vi "SQLite Add Cycle Test.vi"(7 "Test DB Set Up Command":string, 8 "Error In (no error)":errorcluster, 11 "SQLite DB Operator In":refnum<class "SQLite DB Operator.lvclass">) -> (0 "Error Out":errorcluster, 3 "SQLite DB OperatorOut":refnum<class "SQLite DB Operator.lvclass">)   [LabVIEW 2023]
uses:
  Clasess/SQLite DB Operator/SQLite DB Operator.lvclass
  Clasess/DB Records/Expenses Tracker Cycle/Public/Ctrls/Cycle.ctl
  Clasess/DB Records/Expenses Tracker Cycle/Expenses Tracker Cycle.lvclass
  H:/Desktop/LabVIEW/LabView Repo/Expenses-Tracker-DB-Operator/Interfaces/Expenses Tracker Record/Expenses Tracker Record.lvclass
  <vilib>/drjdpowell/SQLite Library/SQL Connection/Execute SQL (1D Cluster).vi
  <vilib>/addons/_JKI Toolkits/Caraya/classes/Test/Test.lvclass
  <vilib>/drjdpowell/SQLite Library/SQLite.lvlib
  H:/Desktop/LabVIEW/LabView Repo/Expenses-Tracker-DB-Operator/Clasess/DB Records/Expenses Tracker Cycle/Expenses Tracker Cycle.lvclass
  <vilib>/drjdpowell/SQLite Library/SQL Connection/Connection.lvclass
  Support/Adding/Add Record Assert Error.vi
  Support/Adding/Add Record Assert Not Error.vi
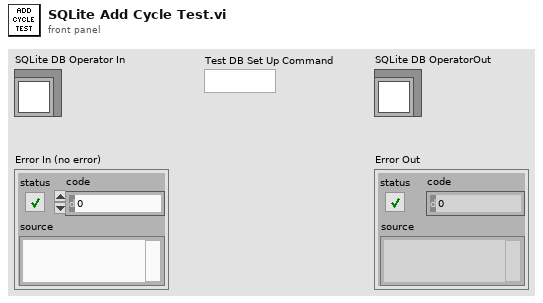
[diagram p1: front panel]
types:
  T1 = typedef "Expenses Tracker Cycle.lvclass/Cycle.ctl" = cluster{"ID":u32, "Name":string, "Day_of_occurence":u8, "Description":string}
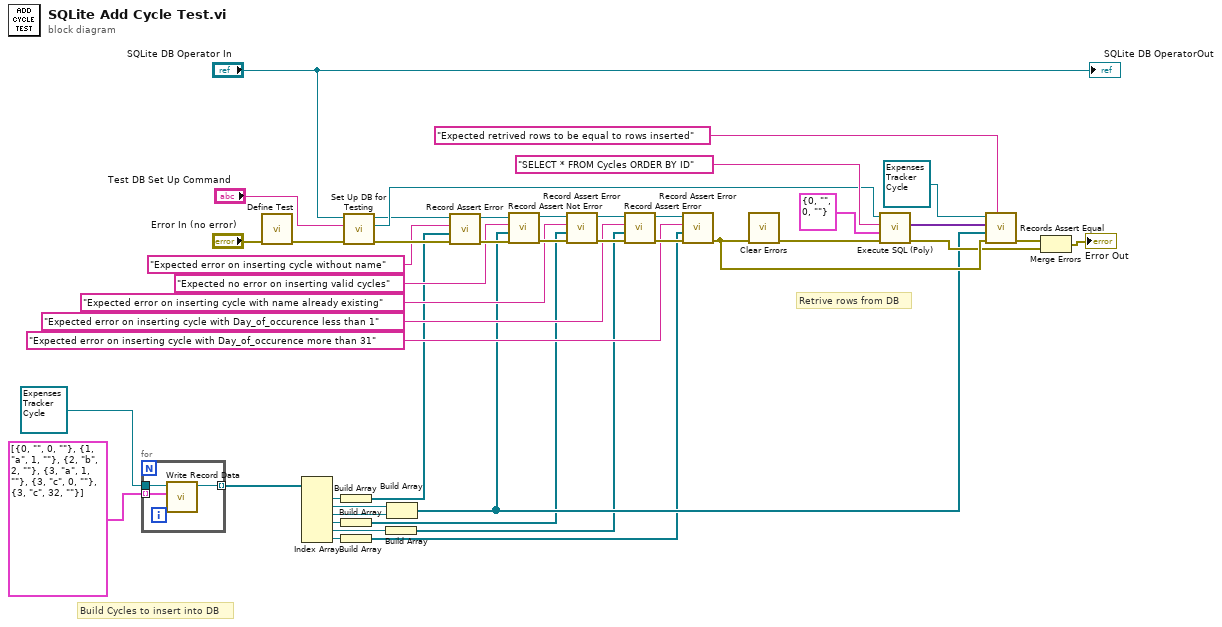
[diagram p0: block diagram]
diagram:
  # "Retrive rows from DB"
  # "Build Cycles to insert into DB"
  n1 = for {
    tunnel: T1[] [{"ID"=0, "Name"="", "Day_of_occurence"=0, "Description"=""}, {"ID"=1, "Name"="a", "Day_of_occurence"=1, "Description"=""}, {"ID"=2, "Name"="b", "Day_of_occurence"=2, "Description"=""}, {"ID"=3, "Name"="a", "Day_of_occurence"=1, "Description"=""}, {"ID"=3, "Name"="c", "Day_of_occurence"=0, "Description"=""}, {"ID"=3, "Name"="c", "Day_of_occurence"=32, "Description"=""}] ("Array") -> [w47] mode=indexing
    tunnel: refnum<class "Expenses Tracker Cycle.lvclass"> refnum ("Expenses Tracker Category") -> [w46]
    tunnel: [w45] -> w41 mode=indexing
    n2 = call-dynamic "Write Record Data.vi"("Record"=w47, "Expenses Tracker Cycle In"=w46) -> ("Expenses Tracker Cycle Out"=w45:refnum<class "Expenses Tracker Cycle.lvclass">)  [unwired: 8 in, 1 out]
  }
  n3 = call <vilib>:"Define Test.vi"("error in (no error)"="Error In (no error)") -> ("error out"=w32:errorcluster)  [unwired: 9 in, 1 out]
  n4 = Index Array(array=w41) -> (element #1=w40:refnum<class "Expenses Tracker Cycle.lvclass">, element #2=w39:refnum<class "Expenses Tracker Cycle.lvclass">, element #3=w38:refnum<class "Expenses Tracker Cycle.lvclass">, element #4=w6:refnum<class "Expenses Tracker Cycle.lvclass">, element #5=w4:refnum<class "Expenses Tracker Cycle.lvclass">, element #6=w35:refnum<class "Expenses Tracker Cycle.lvclass">)  [unwired: 6 in]
  n5 = Build Array(w40) -> (w8:refnum<class "Expenses Tracker Cycle.lvclass">[])
  n6 = Build Array(w6) -> (w5:refnum<class "Expenses Tracker Cycle.lvclass">[])
  n7 = Build Array(w35) -> (w1:refnum<class "Expenses Tracker Cycle.lvclass">[])
  n8 = call "Set Up DB for Testing.vi"("Error In (no error)"=w32, "Test DB Set Up Command"="Test DB Set Up Command", "SQLite DB Operator In"="SQLite DB Operator In") -> ("Error Out"=w31:errorcluster, "SQLite Connection"=w34:refnum<class "Connection.lvclass">, "SQLite DB Operator Out"=w30:refnum<class "SQLite DB Operator.lvclass">)  [unwired: 6 in]
  n9 = Build Array(w4) -> (w3:refnum<class "Expenses Tracker Cycle.lvclass">[])
  n10 = Build Array(w39, w38) -> (w7:refnum<class "Expenses Tracker Cycle.lvclass">[])
  n11 = call-poly "Record Assert Error.vi"("Error In"=w31, "Records"=w8, "Assertion Label"="Expected error on inserting cycle without name" ("Label (VI Title)"), "SQLite DB Operator In"=w30) -> ("Error Out"=w22:errorcluster, "SQLite DB Operator Out"=w21:refnum<class "SQLite DB Operator.lvclass">)  [unwired: 6 in]
  n12 = call-poly "Record Assert Not Error.vi"("Error In"=w22, "Records"=w7, "Assertion Label"="Expected no error on inserting valid cycles" ("Label (VI Title)"), "SQLite DB Operator In"=w21) -> ("Error Out"=w27:errorcluster, "SQLite DB Operator Out"=w28:refnum<class "SQLite DB Operator.lvclass">)  [unwired: 6 in]
  n13 = call-poly "Record Assert Error.vi"("Error In"=w27, "Records"=w5, "Assertion Label"="Expected error on inserting cycle with name already existing" ("Label (VI Title)"), "SQLite DB Operator In"=w28) -> ("Error Out"=w25:errorcluster, "SQLite DB Operator Out"=w26:refnum<class "SQLite DB Operator.lvclass">)  [unwired: 6 in]
  n14 = call-poly "Record Assert Error.vi"("Error In"=w25, "Records"=w3, "Assertion Label"="Expected error on inserting cycle with Day_of_occurence less than 1" ("Label (VI Title)"), "SQLite DB Operator In"=w26) -> ("Error Out"=w23:errorcluster, "SQLite DB Operator Out"=w24:refnum<class "SQLite DB Operator.lvclass">)  [unwired: 6 in]
  n15 = call-poly "Record Assert Error.vi"("Error In"=w23, "Records"=w1, "Assertion Label"="Expected error on inserting cycle with Day_of_occurence more than 31" ("Label (VI Title)"), "SQLite DB Operator In"=w24) -> ("Error Out"=w12:errorcluster)  [unwired: 6 in, 1 out]
  n16 = call <vilib>:"Clear Errors.vi"("error in (no error)"=w12) -> ("error out"=w11:errorcluster)  [unwired: 5 in, 1 out]
  n17 = call-poly <vilib>:"Execute SQL (Poly).vi"("error in (no error)"=w11, "Cluster (or Array of Clusters)"=T1 {"ID"=0, "Name"="", "Day_of_occurence"=0, "Description"=""} ("Cycle"), "SQL"="SELECT * FROM Cycles ORDER BY ID", "SQLite Connection in"=w34) -> ("error out"=w9:errorcluster, "Result Set (Array of Clusters)"=w15:variant[])  [unwired: 5 in, 1 out]
  n18 = call "Records Assert Equal.vi"("Assertion Label"="Expected retrived rows to be equal to rows inserted" ("Label (VI Title)"), "Error In"=w12, "Correct Records"=w7, "Typedef Records"=w15, "Expenses Tracker Record In"=refnum<class "Expenses Tracker Cycle.lvclass"> refnum ("Expenses Tracker Category")) -> ("Error Out"=w10:errorcluster)  [unwired: 6 in]
  n19 = Merge Errors(w10, w9) -> (→"Error Out":errorcluster)
  "SQLite DB OperatorOut" <- "SQLite DB Operator In"
